vi "EnumToString.vi"(10 "Current Station":T1) -> (2 "String":string)   [LabVIEW 2020]
uses:
  Controls/Queue_Control.ctl
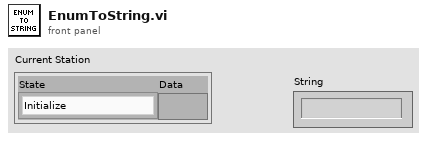
[diagram p1: front panel]
types:
  T1 = typedef "Queue_Control.ctl" = cluster{"State":enum16{"Initialize", "Start", "Next Station", "Under Body Wash", "Bug Remover", "Pre-soak", "High Pressure Wash", "Low Pressure Wash", "Spot Free Rinse", "Tire Shine Foam", "Air Dry", "Exit", "Check Position", "Out of Position", "Stop"}, "Data":variant}
  T2 = enum16{"Initialize", "Start", "Next Station", "Under Body Wash", "Bug Remover", "Pre-soak", "High Pressure Wash", "Low Pressure Wash", "Spot Free Rinse", "Tire Shine Foam", "Air Dry", "Exit", "Check Position", "Out of Position", "Stop"}
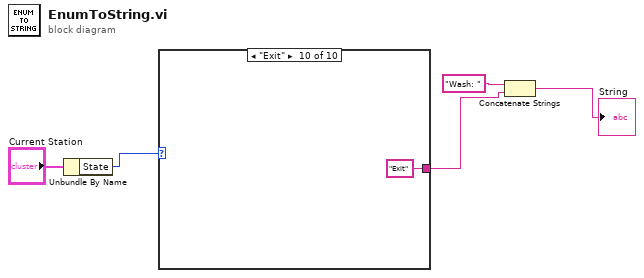
[diagram p0: block diagram]
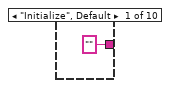
[diagram p2: hidden frame]
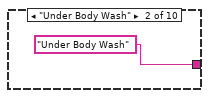
[diagram p3: hidden frame]
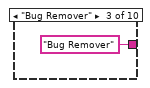
[diagram p4: hidden frame]
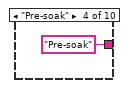
[diagram p5: hidden frame]
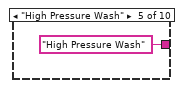
[diagram p6: hidden frame]
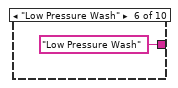
[diagram p7: hidden frame]
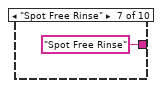
[diagram p8: hidden frame]
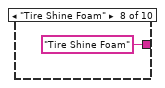
[diagram p9: hidden frame]
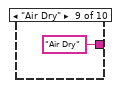
[diagram p10: hidden frame]
diagram:
  n1 = Unbundle By Name("Current Station") -> ("State"=w4:T2)
  n2 = case shown="\"Exit\"" w4 {
    tunnel: ["" ("String") "Under Body Wash" ("String") "Bug Remover" ("String") "Pre-soak" ("String") "High Pressure Wash" ("String") "Low Pressure Wash" ("String") "Spot Free Rinse" ("String") "Tire Shine Foam" ("String") "Air Dry" ("String") "Exit" ("String")] -> w2
    frame "Initialize", Default {
    }
    frame "Under Body Wash" {
    }
    frame "Bug Remover" {
    }
    frame "Pre-soak" {
    }
    frame "High Pressure Wash" {
    }
    frame "Low Pressure Wash" {
    }
    frame "Spot Free Rinse" {
    }
    frame "Tire Shine Foam" {
    }
    frame "Air Dry" {
    }
    frame "Exit" {
    }
  }
  n3 = Concatenate Strings("Wash: " ("string"), w2) -> (→"String":string)
